vi "ex9.vi"() -> ()   [LabVIEW 2022 SP3]
panel:
  out "result text":string
  in  "orginal text":string
  in  "Word":string
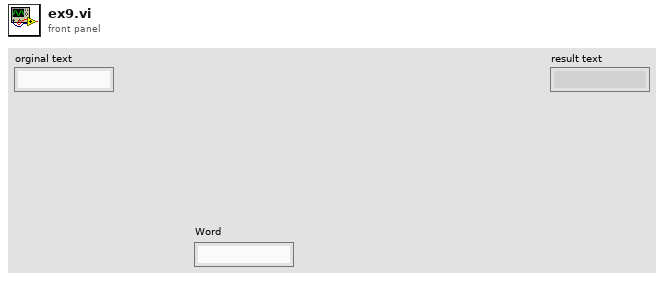
[diagram p1: front panel]
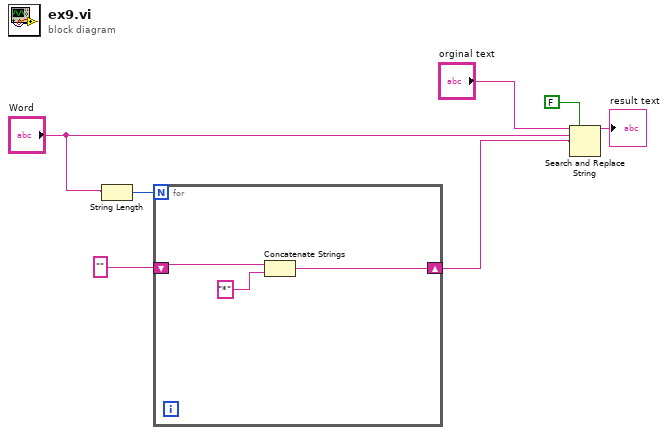
[diagram p0: block diagram]
diagram:
  n1 = String Length(string="Word") -> (length=w4:i32)
  n2 = for {
    N: w4 -> [_]
    shift-right: [w8] -> w1
    shift-left: "" ("Word") -> [w10]
    n3 = Concatenate Strings(w10, "*" ("element")) -> (w8:string)
  }
  n4 = Search and Replace String(replace all?=FALSE ("replace all? (F)"), input string="orginal text", search string="Word", replace string=w1) -> (result string=→"result text":string)  [unwired: 4 in, 3 out]
